vi "ma_ErrorCode2ErrorCluster.vi"(1 "error in (no error)":errorcluster, 2 "subVI Name":string, 3 "Current VI Path":path, 4 "Error Code":i32) -> (0 "error out":errorcluster)   [LabVIEW 2020, in "NI_MABase.lvlib"]
uses:
  NI_MABase.lvlib
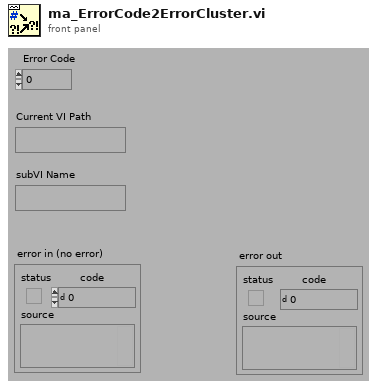
[diagram p1: front panel]
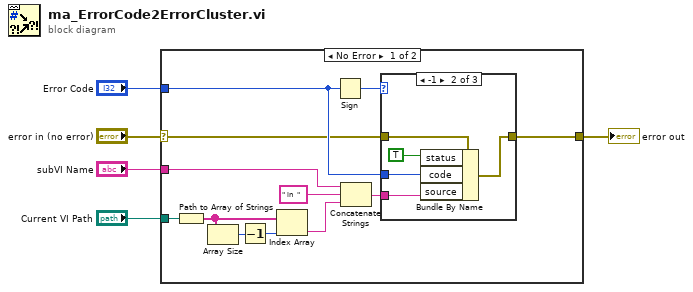
[diagram p0: block diagram]
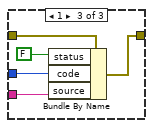
[diagram p3: hidden frame]
diagram:
  n1 = case shown="No Error" "error in (no error)" {
    selector: "error in (no error)" -> [w6 w29]
    tunnel: "Error Code" -> [w16 _]
    tunnel: "Current VI Path" -> [w12 _]
    tunnel: "subVI Name" -> [w11 _]
    tunnel: [w7 w29] -> w2
    frame No Error {
      n2 = Path to Array of Strings(0:w12) -> (2:w15:string[])  [unwired: 1 out]
      n3 = Array Size(array=w15) -> (size(s)=w14:i32)
      n4 = Decrement(x=w14) -> (x-1=w13:i32)
      n5 = Index Array(array=w15, index=w13) -> (element=w9:string)
      n6 = Sign(1:w16) -> (0:w17:i32)
      n7 = Concatenate Strings(w11, " in  " ("Substring"), w9) -> (w8:string)
      n8 = case shown="-1" w17 {
        tunnel: w16 -> [_ w20 w25]
        tunnel: w8 -> [_ w21 w26]
        tunnel: w6 -> [w18 w23 w28]
        tunnel: [w18 w19 w24] -> w7
        frame 0, Default {
        }
        frame -1 {
          n9 = Bundle By Name(cluster=w23, "status"=TRUE ("Bundle Element"), "code"=w20, "source"=w21) -> (w19:errorcluster)
        }
        frame 1 {
          n10 = Bundle By Name(cluster=w28, "status"=FALSE ("Bundle Element"), "code"=w25, "source"=w26) -> (w24:errorcluster)
        }
      }
    }
    frame Error {
    }
  }
  "error out" <- w2
